vi "Command_Joint_Angles.vi"(0 "Side":T2, 1 "node":string, 2 "Arm Angles (degrees)":T1, 3 "error in":errorcluster) -> (6 "error out":errorcluster)   [LabVIEW 2010]
uses:
  <userlib>/ROSforLV_0.1/ROS/Code/SubVIs/BaxterSide.ctl
  <userlib>/ROSforLV_0.1/ROS/Code/SubVIs/BaxterArmsSmall.ctl
panel:
  out "Move Command":string
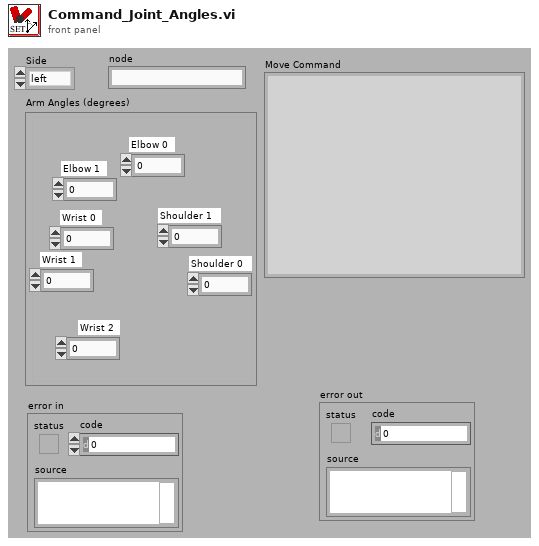
[diagram p1: front panel]
types:
  T1 = typedef "BaxterArmsSmall.ctl" = cluster{"Elbow 0":dbl, "Elbow 1":dbl, "Shoulder 0":dbl, "Shoulder 1":dbl, "Wrist 0":dbl, "Wrist 1":dbl, "Wrist 2":dbl}
  T2 = typedef "BaxterSide.ctl" = enum16{"left", "right"}
  T3 = typedef "_ROSControl.ctl" = cluster{"topic port":u16, "Node":string, "topic":string, "type":string, "node port":u32, "error ":errorcluster, "Direction":T4, "APIs":string[]}
  T4 = typedef "_ROSDirection.ctl" = enum16{"Node", "Publisher", "Subscriber", "Service Client"}
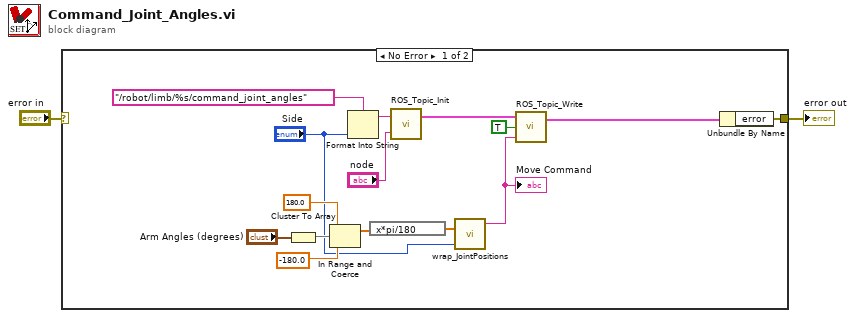
[diagram p0: block diagram]
diagram:
  n1 = case shown="No Error" "error in" {
    selector: "error in" -> [_ w18]
    tunnel: [w17 w18] -> w2
    frame No Error {
      n2 = Cluster To Array(cluster="Arm Angles (degrees)") -> (array=w10:dbl[])
      n3 = In Range and Coerce(upper limit=180.0 ("Elbow 0"), x=w10, lower limit=-180.0 ("Elbow 0")) -> (coerced(x)=w6:dbl[])  [unwired: 1 out]
      n4 = Format Into String(format string="/robot/limb/%s/command_joint_angles" ("topic"), "Side") -> (resulting string=w14:string)  [unwired: 2 in, 1 out]
      n5 = expression code="x*pi/180"(w6) -> (w5:dbl[])
      n6 = call <userlib>:"ROS_Topic_Init.vi"("node"="node", "topic"=w14) -> ("ROS out"=w13:T3)  [unwired: 1 in]
      n7 = call <userlib>:"wrap_JointPositions.vi"("Side"="Side", "Positions"=w5) -> ("msg out"=w7:string)  [unwired: 3 in]
      "Move Command" <- w7
      n8 = call <userlib>:"ROS_Topic_Write.vi"("Msg in"=w7, "Continuous?"=TRUE, "ROS in"=w13) -> ("ROS out"=w12:T3)  [unwired: 1 in]
      n9 = Unbundle By Name(w12) -> ("error"=w17:errorcluster)
    }
    frame Error {
    }
  }
  "error out" <- w2
